vi "new FGGA Serial Data Server & Recordingv4.3.vi"(0 "VISA resource name out":refnum<visa-resource-name>, 11 "error IO":errorcluster) -> ()   [LabVIEW 2014]
uses:
  <vilib>/Platform/TimedLoop/XDataNode/timing_clust.ctl
  <vilib>/Platform/TimedLoop/XDataNode/nitl_modes.ctl
  <vilib>/Platform/TimedLoop/XDataNode/wakeup.ctl
  C:/Program Files (x86)/National Instruments/LabVIEW 2014/examples/Data Communication/Network Streams/Simple Network Streams/support/Network Stream Command.ctl
  <vilib>/Utility/error.llb/whitespace.ctl
  <vilib>/Instr/_visa.llb/VISA Configure Serial Port (Instr).vi
  <vilib>/Utility/tcp.llb/UDP Multicast Write-Only Open.vi
  <vilib>/platform/TimedLoop/XDataNode/XDataNode.xnode
  <vilib>/Platform/TimedLoop/XDataNode/XDNodeRunTimeDep.lvlib
panel:
  out "ASCII_file_out":string
  out "Unix time":u32
  out "FGGA Pump":bool
  out "Flight Number":string
  out "Stop File Write":bool
  out "Default file name":string
  out "MFC":dbl[](array[numeric])
  out "FGGA restart":bool
  out "V4":bool
  out "V3":bool
  out "V2":bool
  out "V1":bool
  out "error out 2":errorcluster
  out "error out":errorcluster
  in  "MFC_1 SLPM set value":dbl
  out "Value Read":string
  out "status":bool
  in  "VISA resource name":refnum<visa-resource-name>="ASRL3::INSTR"
  in  "timeout (10sec) 2":u32=3000
  in  "Clear Display\nErrors":bool
  out "Data Processing":bool
  out "TCP Binary Packet":string
  out "UDP Time Stamp Offset":i32=1
  out "Data String":string
  out "UDP_ACSII_Out":string
  out "Serial error out":errorcluster
  out "SEPTIC TCP Error Out":errorcluster
  out "TCP packet\nSend To SEPTIC":bool
  out "FISH TCP Error Out":errorcluster
  out "TCP packet\nSend To FISH":bool
  out "UDP_Pack_num":u32
  out "UDP_Out Status":bool
  out "UDP_Out_Error Out":errorcluster
  out "Data Array":string[](array[string])
  out "RAW DATA":string
  in  "stop":bool
  out "Number of times \nRead time out":u32
  out "Loop count":i32
  # "Date"
  # "Time"
  # "CH4_wet_ppm"
  # "1"
  # "CO4_wet_ppm_sd"
  # "H2O_ppm"
  # "3"
  # "H2O_ppm_sd"
  # "CO2_wet_ppm"
  # "5"
  # "CO2_wet_ppm_sd"
  # "CH4_dry_ppm"
  # "CH4_dry_ppm_sd"
  # "CO2_dry_ppm"
  # "CO2_dry_ppm_sd"
  # "cell_pressure_torr"
  # "11"
  # "cell_pressure_torr_sd"
  # "13"
  # "cell_temp_degC"
  # "cell_temp_degC_sdev"
  # "ambient(bench)_temp_degC"
  # "15"
  # "ambient(bench)_temp_dedgC_sd"
  # "17"
  # "RDA_us"
  # "RDA_us_sd"
  # "RDB_us"
  # "19"
  # "RDB_us_sd"
  # "Fitflag"
  # "21"
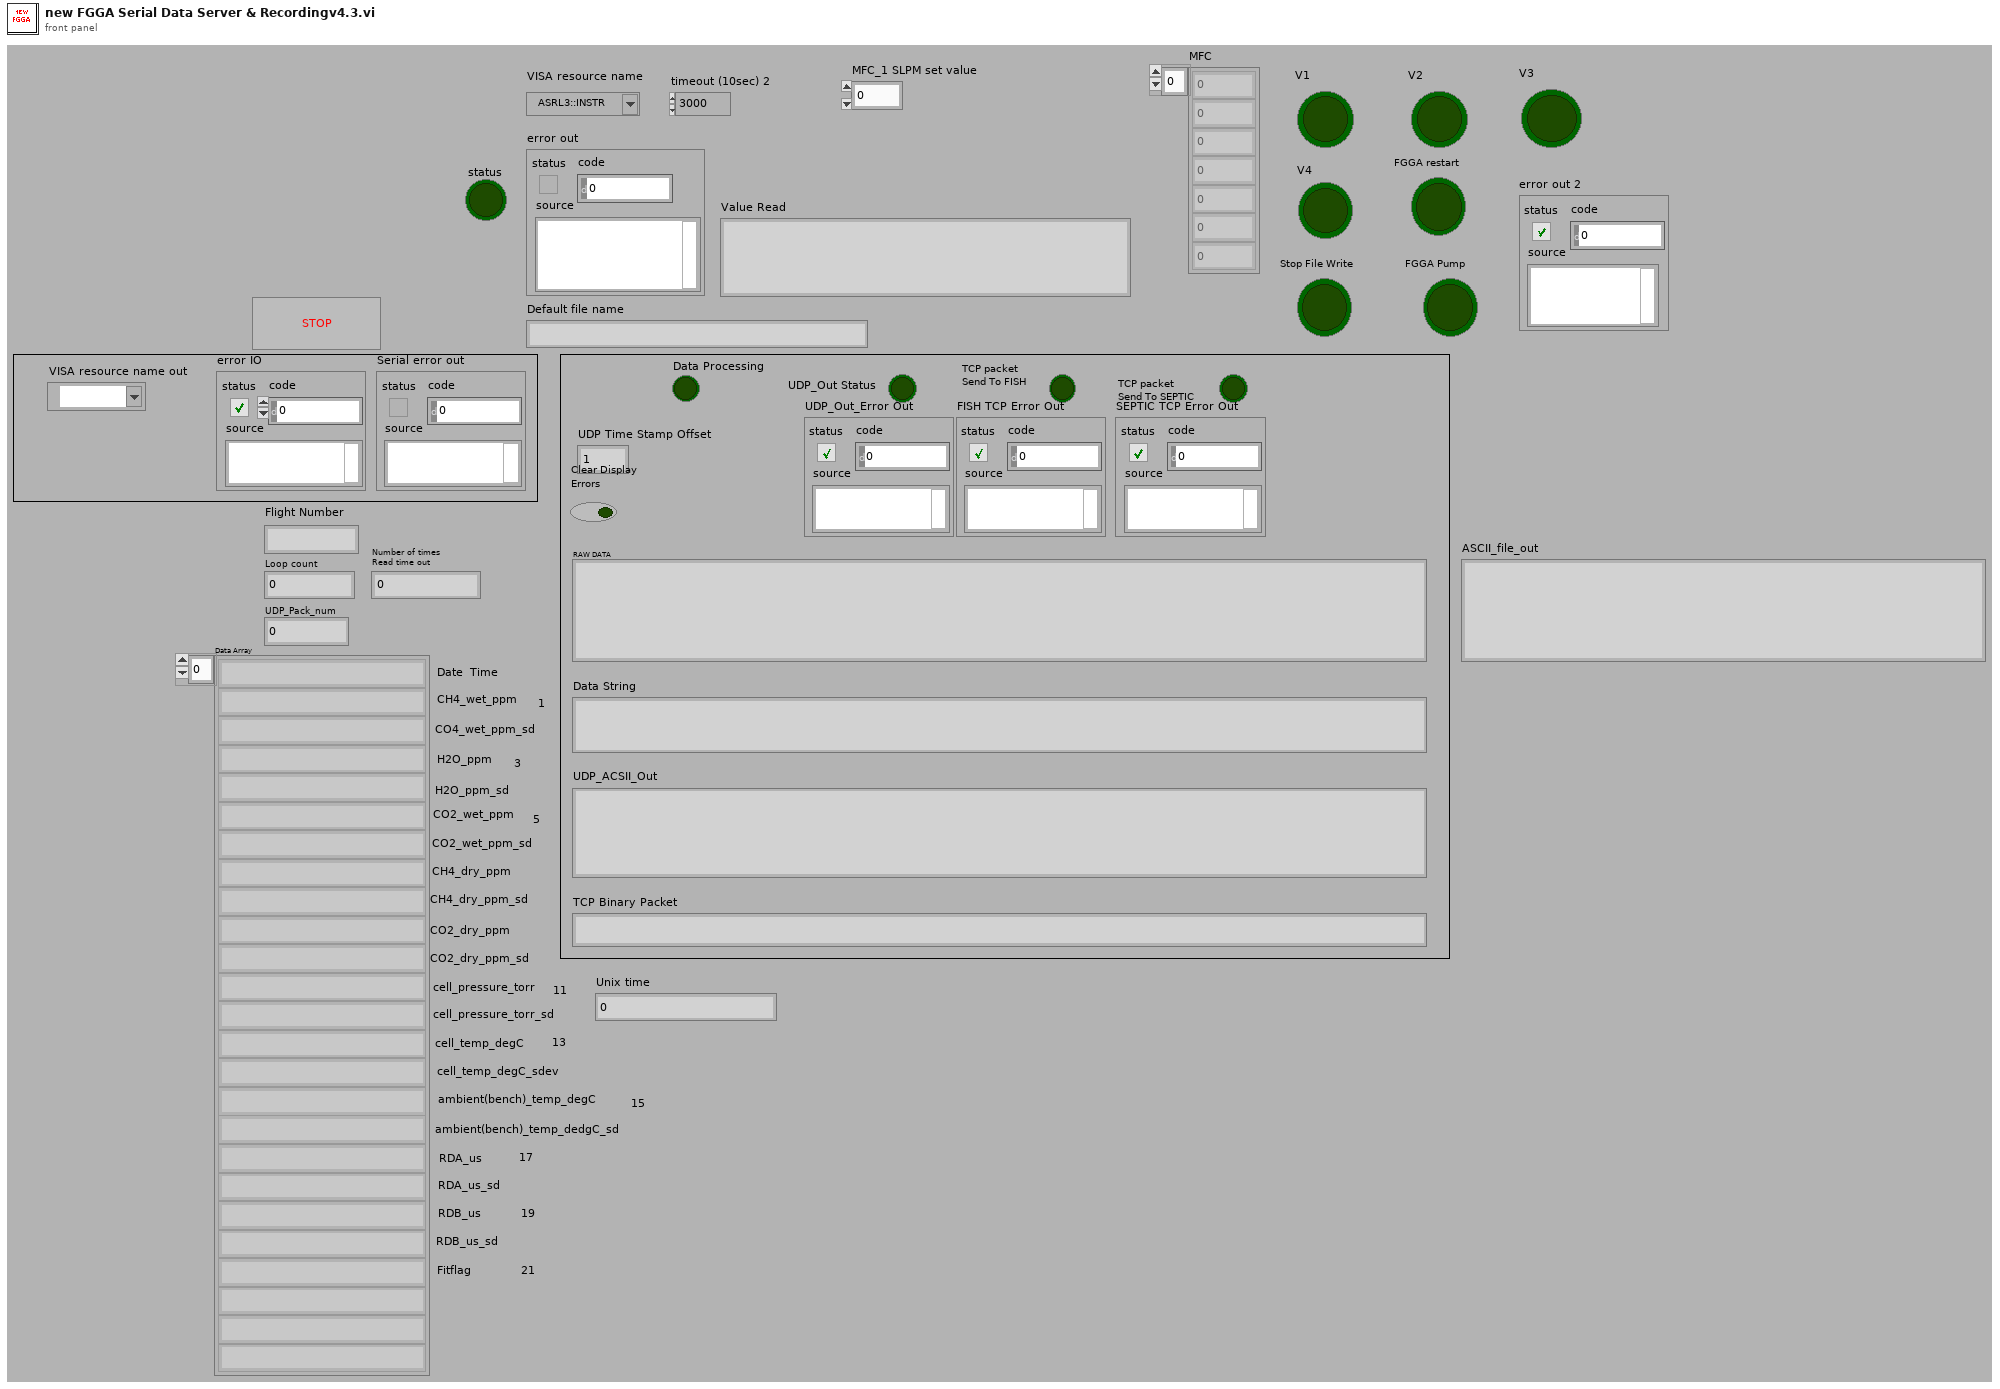
[diagram p1: front panel]
types:
  T1 = typedef "XDNodeRunTimeDep.lvlib/timing_clust.ctl" = cluster{"Expected End [f-1]":u64, "Actual End [f-1]":u64, "Finished Late? [f-1]":bool, "Expected End [i-1]":u64, "Actual End [i-1]":u64, "Finished Late? [i-1]":bool, "Expected Start [i]":u64, "Actual Start [i]":u64, "Expected Start [f]":u64, "Actual Start [f]":u64, "Source Name":string, "Structure Name":string, "Period":i64, "Deadline":i64, "Offset":i64, "Start":i64, "Priority":i32, "Timeout":i32, "Mode":T2, "Wakeup Reason":T3, "Error":errorcluster, "Source Type":string, "Secondary Source Type":string, "Global End Time":u64, "Global Start Time":u64, "Frame Duration":u64, "Iteration Duration":u64, "Assigned CPU":i32, "I/O Scan Engine Mode":u32}
  T2 = typedef "XDNodeRunTimeDep.lvlib/nitl_modes.ctl" = enum32{"No Change", "Process missed periods, maintain original phase", "Discard missed periods, maintain original phase", "Process missed periods, ignore original phase", "Discard missed periods, ignore original phase"}
  T3 = typedef "XDNodeRunTimeDep.lvlib/wakeup.ctl" = enum32{"Normal", "Aborted", "Asynchronous wakeup", "Timing source error", "Timed loop error", "Timeout"}
  T4 = enum16{"open", "replace", "create", "open or create", "replace or create", "replace or create with confirmation"}
  T5 = typedef "Network Stream Command.ctl" = cluster{"Message":string, "Message Data":variant}
  T6 = typedef "whitespace.ctl" = u16
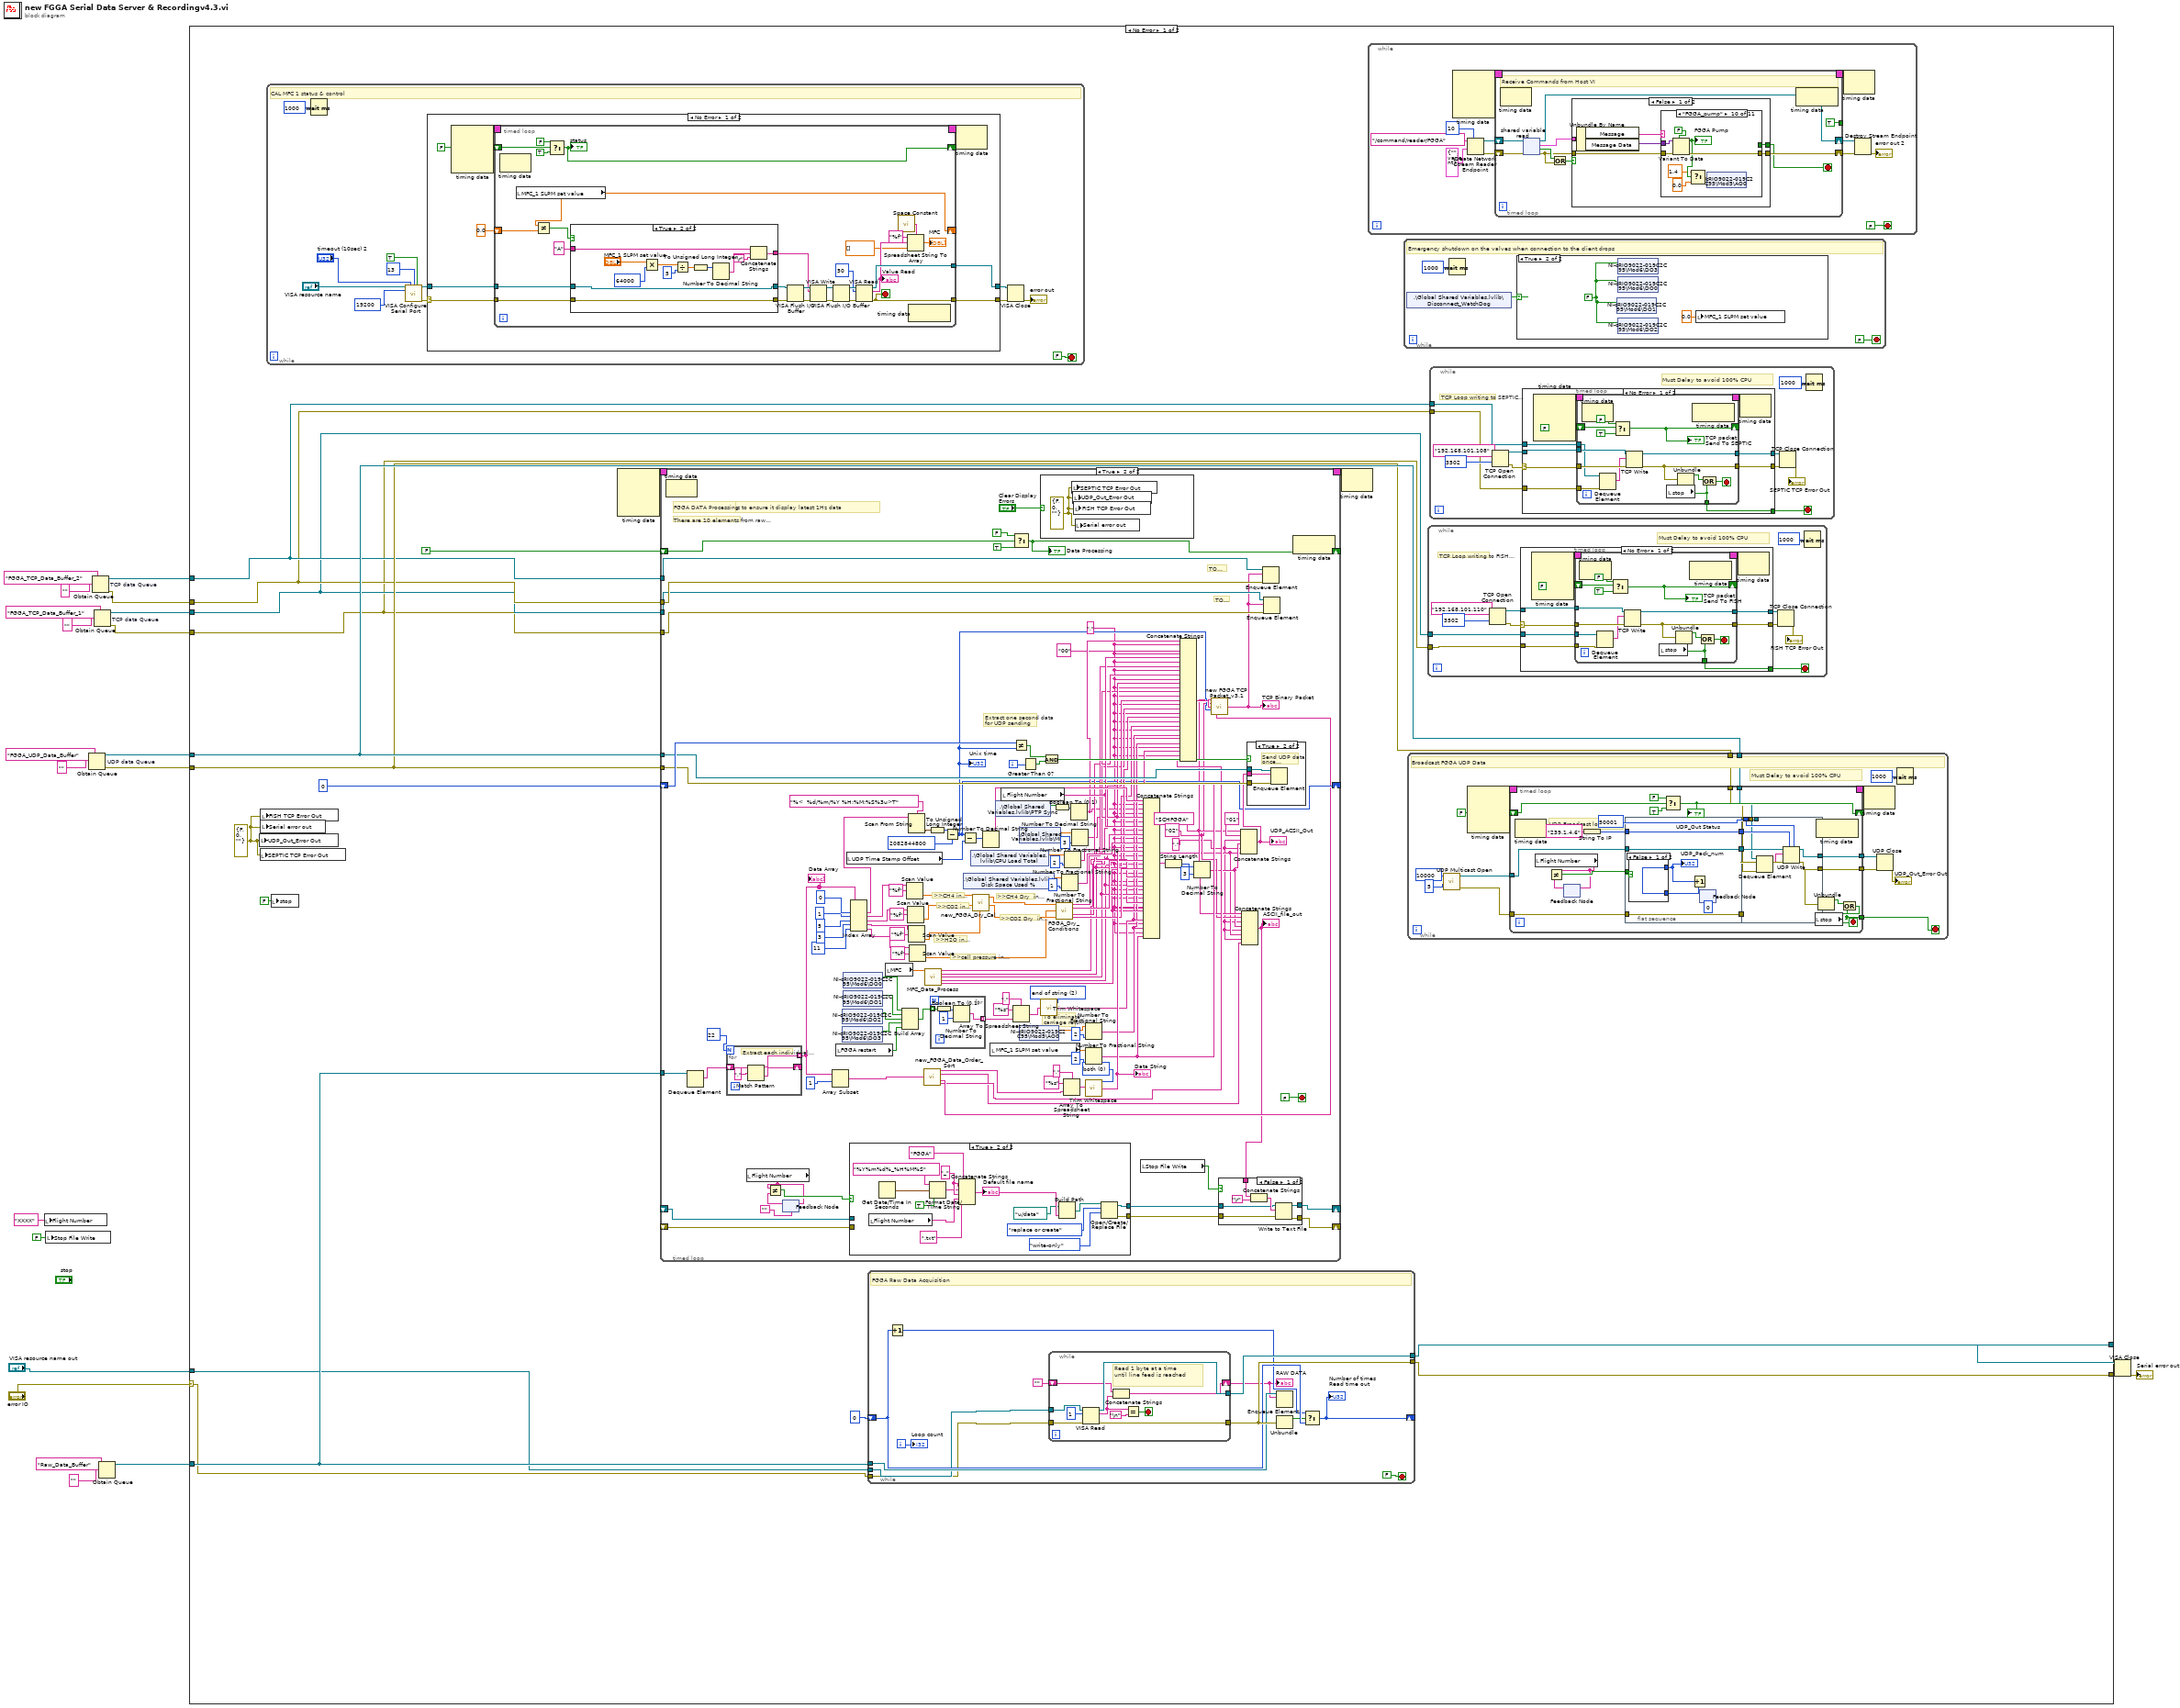
[diagram p0: block diagram]
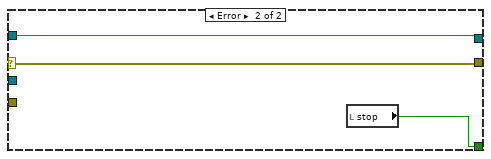
[diagram p2: hidden frame]
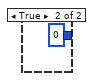
[diagram p3: hidden frame]
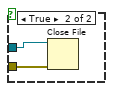
[diagram p5: hidden frame]
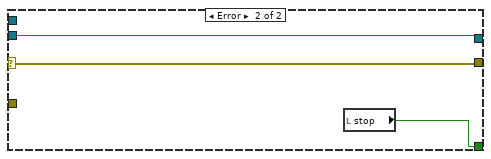
[diagram p8: hidden frame]
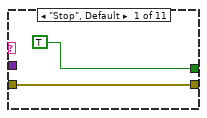
[diagram p10: hidden frame]
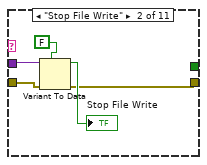
[diagram p11: hidden frame]
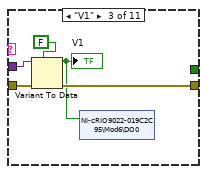
[diagram p12: hidden frame]
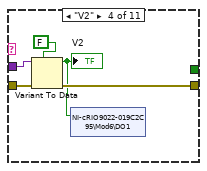
[diagram p13: hidden frame]
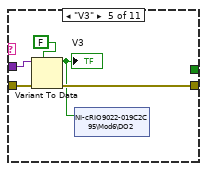
[diagram p14: hidden frame]
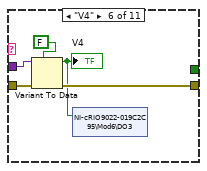
[diagram p15: hidden frame]
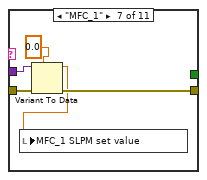
[diagram p16: hidden frame]
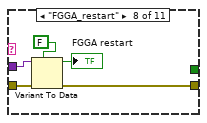
[diagram p17: hidden frame]
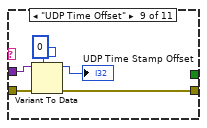
[diagram p18: hidden frame]
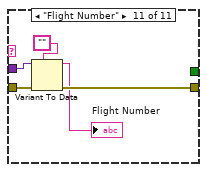
[diagram p19: hidden frame]
diagram:
  n1 = local write "Flight Number"("XXXX" ("Flight Number")) -> ()
  n2 = local write "Stop File Write"(FALSE ("Stop File Write")) -> ()
  n3 = Obtain Queue "UDP data Queue"(name (unnamed)="FGGA_UDP_Data_Buffer", element data type="") -> (queue out=w14:refnum<queue>, error out=w13:errorcluster)  [unwired: 3 in, 1 out]
  n4 = Obtain Queue "TCP data Queue"(name (unnamed)="FGGA_TCP_Data_Buffer_2", element data type="") -> (queue out=w8:refnum<queue>, error out=w7:errorcluster)  [unwired: 3 in, 1 out]
  n5 = Obtain Queue "TCP data Queue"(name (unnamed)="FGGA_TCP_Data_Buffer_1", element data type="") -> (queue out=w6:refnum<queue>, error out=w5:errorcluster)  [unwired: 3 in, 1 out]
  n6 = Obtain Queue(name (unnamed)="Raw_Data_Buffer", element data type="") -> (queue out=w20:refnum<queue>)  [unwired: 3 in, 2 out]
  n7 = case shown="No Error" "error IO" {
    selector: "error IO" -> [w27 w538]
    tunnel: "VISA resource name out" -> [w28 w539]
    tunnel: [w39 w539] -> w17
    tunnel: [w40 w538] -> w18
    tunnel: w20 -> [w38 _]
    tunnel: w14 -> [w36 _]
    tunnel: w13 -> [w35 _]
    tunnel: w8 -> [w34 _]
    tunnel: w7 -> [w33 _]
    tunnel: w6 -> [w32 _]
    tunnel: w5 -> [w31 _]
    frame No Error {
      w24 = errorcluster {"status"=FALSE, "code"=0, "source"=""} ("UDP Error Out")
      n8 = local write "UDP_Out_Error Out"(w24) -> ()
      n9 = local write "SEPTIC TCP Error Out"(w24) -> ()
      n10 = local write "FISH TCP Error Out"(w24) -> ()
      n11 = local write "Serial error out"(w24) -> ()
      n12 = while {
        stop <- FALSE stop-if-true
        # "CAL MFC 1 status & control"
        n13 = Wait (ms)(milliseconds to wait=u32 1000) -> ()  [unwired: 1 out]
        n14 = call-poly "VISA Configure Serial Port"("VISA resource name"="VISA resource name", "timeout (10sec)"="timeout (10sec) 2", "termination char\n(0xA = '\\n' = LF)"=u8 13 ("termination char\n(0xA = '\\n' = LF)"), "Enable Termination\nChar (T)"=TRUE ("Enable Termination\nChar (T)"), "baud rate (9600)"=u32 19200) -> ("VISA resource name out"=w479:refnum<visa-resource-name>, "error out"=w475:errorcluster)  [unwired: 9 in]
        n15 = case shown="No Error" w475 {
          selector: w475 -> [w486 w536]
          tunnel: w479 -> [w487 w537]
          tunnel: [w485 w537] -> w478
          tunnel: [w484 w536] -> w477
          frame No Error {
            n16 = node-c288() -> (w482:T1)  [unwired: 4 in]
            n17 = timed-loop {
              tunnel: w487 -> [w510]
              tunnel: w486 -> [w508]
              tunnel: [w501] -> w485
              tunnel: [w496] -> w484
              shift-right: [w497] -> _
              shift-left: FALSE -> [w500]
              timing: w482 -> [_]
              timing-out: [_] -> w481
              shift-right: [w488] -> _
              shift-left: 0.0 -> [w490]
              stop <- w496 stop-if-true
              n18 = node-c288() -> ()  [unwired: 1 in, 1 out]
              n19 = local read "MFC_1 SLPM set value"() -> (w488:dbl)
              n20 = Not Equal?(x=w488, y=w490) -> (x != y?=w489:bool)
              n21 = Select(t=FALSE, s=w500, f=TRUE) -> (s? t:f=w497:bool)
              "status" <- w497
              n22 = case shown="True" w489 {
                tunnel: w510 -> [w518 w533]
                tunnel: [w518 w533] -> w509
                tunnel: w508 -> [w517 w532]
                tunnel: [w517 w532] -> w507
                tunnel: "A" -> [w521 w525]
                tunnel: [w519 w522] -> w505
                frame False {
                  n23 = Concatenate Strings(w521, "\r") -> (w519:string)
                }
                frame True {
                  n24 = Multiply(x="MFC_1 SLPM set value", y=u32 64000) -> (x*y=w529:dbl)
                  n25 = Divide(x=w529, y=u32 5) -> (x/y=w527:dbl)
                  n26 = To Unsigned Long Integer(number=w527) -> (unsigned 32bit integer=w526:u32)
                  n27 = Number To Decimal String(number=w526) -> (decimal integer string=w524:string)  [unwired: 1 in]
                  n28 = Concatenate Strings(w525, w524, "\r") -> (w522:string)
                }
              }
              n29 = VISA Flush I/O Buffer(VISA resource name=w509, error in (no error)=w507) -> (VISA resource name out=w512:refnum<visa-resource-name>, error out=w511:errorcluster)  [unwired: 1 in]
              n30 = VISA Write(VISA resource name=w512, write buffer=w505, error in (no error)=w511) -> (VISA resource name out=w504:refnum<visa-resource-name>, error out=w503:errorcluster)  [unwired: 1 out]
              n31 = VISA Flush I/O Buffer(VISA resource name=w504, error in (no error)=w503) -> (VISA resource name out=w514:refnum<visa-resource-name>, error out=w513:errorcluster)  [unwired: 1 in]
              n32 = VISA Read(VISA resource name=w514, byte count=u32 50, error in (no error)=w513) -> (VISA resource name out=w501:refnum<visa-resource-name>, read buffer=w495:string, error out=w496:errorcluster)  [unwired: 1 out]
              "Value Read" <- w495
              n33 = call <vilib>:"Space Constant.vi"() -> ("String"=w494:string)
              n34 = Spreadsheet String To Array(delimiter (Tab)=w494, format string="%f", spreadsheet string=w495, array type (2D Dbl)=dbl[] []) -> (array=→"MFC":dbl[])
              n35 = node-c288() -> ()  [unwired: 1 in, 1 out]
            }
            n36 = node-c288(w481) -> ()  [unwired: 1 out]
          }
          frame Error {
          }
        }
        n37 = VISA Close(VISA resource name=w478, error in (no error)=w477) -> (error out=→"error out":errorcluster)
      }
      n38 = local write "stop"(FALSE ("stop")) -> ()
      n39 = node-c288() -> (w26:T1)  [unwired: 4 in]
      n40 = timed-loop {
        timing: w26 -> [_]
        timing-out: [_] -> w25
        tunnel: w38 -> [w290]
        tunnel: w36 -> [w258]
        tunnel: w35 -> [w257]
        shift-right: [w185] -> _
        shift-left: u32 0 -> [w261]
        tunnel: w34 -> [w256]
        tunnel: w33 -> [w255]
        tunnel: w32 -> [w254]
        tunnel: w31 -> [w253]
        shift-right: [w249] -> _
        shift-left: FALSE -> [w252]
        shift-right: [w238] -> _
        shift-left: _ -> [w230]
        shift-right: [w228] -> _
        shift-left: _ -> [w229]
        i -> [w260]
        stop <- FALSE stop-if-true
        w202 = T6 2 items=["both", "start of string", "end of string"] ("location (both)")
        w178 = ","
        w279 = T6 0 items=["both", "start of string", "end of string"] ("location (both)")
        w166 = ","
        w170 = "02"
        w171 = "$CHFGGA"
        # "To eliminate\ncarriage return"
        # ">>cell pressure in torr>>"
        # "There are 10 elements from raw packet"
        # "TO SEPTIC"
        # "TO FISH"
        # "Extract one second data\nfor UDP sending"
        # ">>CO2 Dry  in ppm>>"
        # ">>CH4 Dry  in ppb>>"
        # ">>H2O in ppm>>"
        # ">>CO2 in ppm>>"
        # ">>CH4 in ppm>>"
        # "Loop Time is 500msec to ensure it display latest 1Hz data"
        # "FGGA DATA Processing"
        n41 = node-c288() -> ()  [unwired: 1 in, 1 out]
        n42 = Dequeue Element(queue=w290) -> (element=w248:string)  [unwired: 2 in, 3 out]
        n43 = for {
          N: 22 -> [_]
          shift-right: [w327] -> _
          shift-left: w248 -> [w325]
          tunnel: [w326] -> w284 mode=indexing
          # "Extract each individual param"
          n44 = Match Pattern(string=w325, regular expression=",") -> (before substring=w326:string, after substring=w327:string)  [unwired: 1 in, 2 out]
        }
        "Data Array" <- w284
        n45 = local read "Flight Number"() -> (w227:string)
        n46 = feedback #1("" ("Flight Number")) -> (w235:string)
        n47 = Not Equal?(x=w227, y=w235) -> (x != y?=w233:bool)
        n48 = feedback-in #1(w227) -> ()
        n49 = Array Subset(array=w284, index=1) -> (w176:string[])  [unwired: 1 in]
        n50 = local read "FGGA restart"() -> (w212:bool)
        n51 = shared-variable "NI-cRIO9022-019C2C95\\Mod6\\DO2"() -> (w218:bool)  [unwired: 1 in, 1 out]
        n52 = shared-variable "NI-cRIO9022-019C2C95\\Mod6\\DO3"() -> (w217:bool)  [unwired: 1 in, 1 out]
        n53 = shared-variable "NI-cRIO9022-019C2C95\\Mod6\\DO0"() -> (w220:bool)  [unwired: 1 in, 1 out]
        n54 = shared-variable "NI-cRIO9022-019C2C95\\Mod6\\DO1"() -> (w219:bool)  [unwired: 1 in, 1 out]
        n55 = local read "UDP Time Stamp Offset"() -> (w201:i32)
        n56 = case shown="True" w233 {
          tunnel: [w296 w298] -> w232
          tunnel: [w295 w297] -> w231
          tunnel: w230 -> [w296 _]
          tunnel: w229 -> [w295 _]
          frame False {
          }
          frame True {
            w304 = "_" ("string")
            n57 = local read "Flight Number"() -> (w311:string)
            n58 = Get Date/Time In Seconds() -> (seconds since 1Jan1904=w299:timestamp)
            n59 = Format Date/Time String(time format string (%c)="%Y%m%d%_%H%M%S", seconds (now)=w299, UTC format=TRUE) -> (date/time string=w301:string)
            n60 = Concatenate Strings("FGGA" ("string"), w304, w301, w304, w311, ".txt" ("string")) -> (w306:string)
            "Default file name" <- w306
            n61 = Build Path(base path=path "u:/data", name or relative path=w306) -> (appended path=w310:path)
            n62 = Open/Create/Replace File(file path (use dialog)=w310, operation (0:open)=T4."replace or create", access (0:read/write)=enum16{"read/write", "read-only", "write-only"}."write-only") -> (refnum out=w298:refnum<file>, error out=w297:errorcluster)  [unwired: 3 in, 1 out]
          }
        }
        n63 = Index Array(array=w284, index #1=0 ("index"), index #2=1 ("index"), index #3=5 ("index"), index #4=3 ("index"), index #5=11 ("index")) -> (element #1=w179:string, element #2=w184:string, element #3=w183:string, element #4=w182:string, element #5=w181:string)
        n64 = local read "MFC"() -> (w239:dbl[])
        n65 = Build Array(w220, w219, w218, w217, w212) -> (w216:bool[])
        n66 = Scan Value(string=w184, format string="%f") -> (value=w270:dbl)  [unwired: 1 in, 1 out]
        n67 = Scan Value(string=w183, format string="%f") -> (value=w269:dbl)  [unwired: 1 in, 1 out]
        n68 = Scan From String(format string="%<  %d/%m/%Y %H:%M:%S%3u>T", input string=w179) -> (output 1=w266:timestamp)  [unwired: 3 in, 3 out]
        n69 = Scan Value(string=w182, format string="%f") -> (value=w240:dbl)  [unwired: 1 in, 1 out]
        n70 = Scan Value(string=w181, format string="%f") -> (value=w241:dbl)  [unwired: 1 in, 1 out]
        n71 = call "new_FGGA_Data_Order_Sort.vi"("Data In"=w176) -> ("UDP Data Out"=w175:string[], "ASCII Ambient(bench)_temp"=w165:string, "TCP Data Out"=w174:string[], "TCP Ambient(bench)_temp"=w173:string)  [unwired: 11 in]
        n72 = call "MFC_Data_Process.vi"("MFC"=w239) -> ("MFC Absolute Pressure"=w196:string, "MFC Temperature"=w195:string, "MFC Volumetric Flow"=w194:string, "MFC Mass Flow"=w193:string, "MFC Set Point"=w192:string)  [unwired: 10 in]
        n73 = To Unsigned Long Integer(number=w266) -> (unsigned 32bit integer=w267:u32)
        n74 = for {
          tunnel: w216 -> [w293] mode=indexing
          tunnel: [w292] -> w213 mode=indexing
          n75 = Boolean To (0,1)(Boolean=w293) -> (0, 1=w294:i16)
          n76 = Number To Decimal String(number=w294, width (-)=i16 1) -> (decimal integer string=w292:string)
        }
        n77 = Subtract(x=w267, y=u32 2082844800) -> (x-y=w185:u32)
        "Unix time" <- w185
        n78 = Subtract(x=w185, y=w201) -> (x-y=w264:u32)
        n79 = shared-variable ".\\Global Shared Variables.lvlib\\Disk Space Used %"() -> (w205:dbl)  [unwired: 1 in, 1 out]
        n80 = shared-variable ".\\Global Shared Variables.lvlib\\CPU Load Total"() -> (w226:dbl)  [unwired: 1 in, 1 out]
        n81 = call "new_FGGA_Dry_Cal.vi"("H2O"=w240, "CO2_Wet"=w269, "CH4_Wet"=w270) -> ("CO2_Dry"=w243:dbl, "CH4_Dry"=w245:dbl)  [unwired: 7 in]
        n82 = Number To Decimal String(number=w264) -> (decimal integer string=w265:string)  [unwired: 1 in]
        n83 = local read "MFC_1 SLPM set value"() -> (w208:dbl)
        n84 = shared-variable ".\\Global Shared Variables.lvlib\\PTP Sync"() -> (w221:bool)  [unwired: 1 in, 1 out]
        n85 = local read "Flight Number"() -> (w200:string)
        n86 = Array To Spreadsheet String(delimiter (Tab)=",", array=w213, 3:"%s" ("format string")) -> (spreadsheet string=w203:string)
        n87 = Select(t=FALSE, s=w252, f=TRUE) -> (s? t:f=w249:bool)
        "Data Processing" <- w249
        n88 = Not Equal?(x=w261, y=w185) -> (x != y?=w262:bool)
        n89 = shared-variable ".\\Global Shared Variables.lvlib\\MFM"() -> (w224:dbl)  [unwired: 1 in, 1 out]
        n90 = shared-variable "NI-cRIO9022-019C2C95\\Mod5\\AO0"() -> (w210:dbl)  [unwired: 1 in, 1 out]
        n91 = Greater Than 0?(x=w260) -> (x > 0?=w263:bool)
        n92 = case shown="True" "Clear Display\nErrors" {
          frame False {
          }
          frame True {
            w321 = errorcluster {"status"=FALSE, "code"=0, "source"=""} ("UDP Error Out")
            n93 = local write "SEPTIC TCP Error Out"(w321) -> ()
            n94 = local write "UDP_Out_Error Out"(w321) -> ()
            n95 = local write "FISH TCP Error Out"(w321) -> ()
            n96 = local write "Serial error out"(w321) -> ()
          }
        }
        n97 = call <vilib>:"Trim Whitespace.vi"("string"=w203, "location (both)"=w202) -> ("trimmed string"=w191:string)
        n98 = Compound Arithmetic op=AND(w262, w263) -> (w259:bool)
        n99 = Boolean To (0,1)(Boolean=w221) -> (0, 1=w222:i16)
        n100 = call "FGGA_Dry_Conditions.vi"("CH4_Dry"=w245, "Pressure"=w241, "CO2_Dry"=w243) -> ("CH4_Dry_TCP"=w199:string, "CH4_Dry_UDP"=w247:string, "CO2_Dry_TCP"=w198:string, "CO2_Dry_UDP"=w246:string)  [unwired: 9 in]
        n101 = Number To Fractional String(number=w205, precision (6)=i16 1) -> (F-format string=w204:string)  [unwired: 2 in]
        n102 = Array To Spreadsheet String(delimiter (Tab)=",", array=w175, 3:"%s" ("format string")) -> (spreadsheet string=w278:string)
        n103 = Number To Fractional String(number=w226, precision (6)=i16 2) -> (F-format string=w207:string)  [unwired: 2 in]
        n104 = Number To Decimal String(number=w222) -> (decimal integer string=w187:string)  [unwired: 1 in]
        n105 = Number To Fractional String(number=w224, precision (6)=i16 3) -> (F-format string=w197:string)  [unwired: 2 in]
        n106 = Number To Fractional String(number=w210, precision (6)=i16 2) -> (F-format string=w190:string)  [unwired: 2 in]
        n107 = Number To Fractional String(number=w208, precision (6)=i16 2) -> (F-format string=w189:string)  [unwired: 2 in]
        n108 = call <vilib>:"Trim Whitespace.vi"("string"=w278, "location (both)"=w279) -> ("trimmed string"=w277:string)
        "Data String" <- w277
        n109 = local read "Stop File Write"() -> (w236:bool)
        n110 = Concatenate Strings(w265, w178, w187, w178, w197, w178, w200, w178, w207, w178, w204, w178, w277, w178, w247, w178, w246, w178, w196, w178, w195, w178, w194, w178, w193, w178, w192, w178, w191, w178, w190, w178, w189) -> (w168:string)
        n111 = String Length(string=w168) -> (length=w287:i32)
        n112 = Concatenate Strings(w187, w178, "00", w178, w200, w178, w199, w178, w198, w178, w197, w178, w196, w178, w195, w178, w194, w178, w193, w178, w192, w178, w191, w178, w190, w178, w189, w178, w173) -> (w188:string)
        n113 = Number To Decimal String(number=w287, width (-)=i16 3) -> (decimal integer string=w169:string)
        n114 = call "new FGGA TCP Packet_v3.1.vi"("ID"=w171, "Version"=w170, "TCP Packet In"=w188, "utc_time"=w185, "Data Array"=w174) -> ("TCP Binary Packet"=w177:string)  [unwired: 10 in]
        "TCP Binary Packet" <- w177
        n115 = Concatenate Strings(w171, "01", w166, w169, w166, w168) -> (w237:string)
        "UDP_ACSII_Out" <- w237
        n116 = Concatenate Strings(w171, w170, w166, w169, w166, w168, w166, w165) -> (w167:string)
        "ASCII_file_out" <- w167
        n117 = case shown="False" w236 {
          tunnel: w167 -> [w318 _]
          tunnel: [w315 _] -> w238
          tunnel: w232 -> [w314 w320]
          tunnel: w231 -> [w313 w319]
          tunnel: [w312 _] -> w228
          frame False {
            n118 = Concatenate Strings(w318, "\r") -> (w316:string)
            n119 = Write to Text File(file (use dialog)=w314, text=w316, error in=w313) -> (refnum out=w315:refnum<file>, error out=w312:errorcluster)  [unwired: 2 out]
          }
          frame True {
            n120 = Close File(refnum=w320, error in=w319) -> ()  [unwired: 2 out]
          }
        }
        n121 = case shown="True" w259 {
          tunnel: w237 -> [_ w324]
          tunnel: w258 -> [_ w323]
          tunnel: w257 -> [_ w322]
          frame False {
          }
          frame True {
            # "Send UDP data once\na second"
            n122 = Enqueue Element(queue=w323, element=w324, error in (no error)=w322) -> ()  [unwired: 1 in, 3 out]
          }
        }
        n123 = Enqueue Element(queue=w256, element=w177, error in (no error)=w255) -> ()  [unwired: 1 in, 3 out]
        n124 = Enqueue Element(queue=w254, element=w177, error in (no error)=w253) -> ()  [unwired: 1 in, 3 out]
        n125 = node-c288() -> ()  [unwired: 1 in, 1 out]
      }
      n126 = while {
        tunnel: w28 -> [w42]
        tunnel: w27 -> [w41]
        tunnel: [w53] -> w40
        shift-right: [w49] -> _
        shift-left: u32 0 -> [w50]
        tunnel: [w52] -> w39
        tunnel: w38 -> [w47]
        i -> [w51]
        stop <- FALSE stop-if-true
        # "FGGA Raw Data Acquisition"
        n127 = Increment(x=w50) -> (x+1=w48:u32)
        n128 = while {
          tunnel: [w63] -> w52
          tunnel: [w62] -> w53
          tunnel: w42 -> [w61]
          tunnel: w41 -> [w60]
          shift-right: [w58] -> w44
          shift-left: "" -> [w59]
          stop <- w55 stop-if-true
          # "Read 1 byte at a time \nuntil line feed is reached"
          n129 = VISA Read(VISA resource name=w61, byte count=u32 1, error in (no error)=w60) -> (VISA resource name out=w63:refnum<visa-resource-name>, read buffer=w57:string, error out=w62:errorcluster)  [unwired: 1 out]
          n130 = Concatenate Strings(w59, w57) -> (w58:string)
          n131 = Equal?(x=w57, y="\n") -> (x = y?=w55:bool)
        }
        "RAW DATA" <- w44
        n132 = Enqueue Element(queue=w47, element=w44) -> ()  [unwired: 2 in, 3 out]
        n133 = Unbundle(w53) -> ("status"=w46:bool)  [unwired: 2 out]
        n134 = Select(t=w48, s=w46, f=w50) -> (s? t:f=w49:u32)
        "Number of times \nRead time out" <- w49
        "Loop count" <- w51
      }
      n135 = node-c288(w25) -> ()  [unwired: 1 out]
      n136 = while {
        stop <- FALSE stop-if-true
        n137 = node-c288() -> (w381:T1)  [unwired: 4 in]
        n138 = Create Network Stream Reader Endpoint(7:10 ("reader buffer size"), 9:T5 {"Message"="", "Message Data"=variant} ("Message Cluster"), 11:"/command/reader/FGGA" ("reader url")) -> (0:w386:errorcluster, 3:w387:refnum<k21>)  [unwired: 4 in]
        n139 = timed-loop "Host->Target Command Reader" {
          shift-right: [w397] -> w384
          shift-left: w386 -> [w400]
          shift-right: [w398] -> w383
          shift-left: w387 -> [w399]
          tunnel: [TRUE] -> _
          timing: w381 -> [_]
          timing-out: [_] -> w380
          stop <- w391 stop-if-true
          # "Receive Commands from Host VI"
          n140 = node-c288() -> ()  [unwired: 1 in, 1 out]
          n141 = shared-variable-read(w399, w400) -> (w398:refnum<k21>, w393:errorcluster, w395:bool, w396:T5)  [unwired: 1 in]
          n142 = Or(x=w395, y=w393) -> (x .or. y?=w394:bool)
          n143 = case shown="False" w394 {
            selector: w394 -> [_ w464]
            tunnel: w393 -> [w408 w465]
            tunnel: [w407 w465] -> w397
            tunnel: w396 -> [w405 _]
            tunnel: [w406 w464] -> w391
            frame False {
              n144 = Unbundle By Name(w405) -> ("Message"=w404:string, "Message Data"=w403:variant)
              n145 = case shown="\"FGGA_pump\"" w404 {
                tunnel: w408 -> [w410 w415 w420 w425 w430 w435 w440 w445 w450 w458 w463]
                tunnel: [w410 w411 w419 w424 w429 w434 w439 w444 w449 w457 w462] -> w407
                tunnel: w403 -> [_ w414 w418 w423 w428 w433 w438 w443 w448 w456 w461]
                tunnel: [TRUE _ _ _ _ _ _ _ _ _ _] -> w406
                frame "Stop", Default {
                }
                frame "Stop File Write" {
                  n146 = Variant To Data(error in=w415, type=FALSE, Variant=w414) -> (data=→"Stop File Write":bool, error out=w411:errorcluster)
                }
                frame "V1" {
                  n147 = Variant To Data(error in=w420, type=FALSE, Variant=w418) -> (data=w416:bool, error out=w419:errorcluster)
                  "V1" <- w416
                  n148 = shared-variable "NI-cRIO9022-019C2C95\\Mod6\\DO0"(w416) -> ()  [unwired: 1 in, 1 out]
                }
                frame "V2" {
                  n149 = Variant To Data(error in=w425, type=FALSE, Variant=w423) -> (data=w421:bool, error out=w424:errorcluster)
                  "V2" <- w421
                  n150 = shared-variable "NI-cRIO9022-019C2C95\\Mod6\\DO1"(w421) -> ()  [unwired: 1 in, 1 out]
                }
                frame "V3" {
                  n151 = Variant To Data(error in=w430, type=FALSE, Variant=w428) -> (data=w426:bool, error out=w429:errorcluster)
                  "V3" <- w426
                  n152 = shared-variable "NI-cRIO9022-019C2C95\\Mod6\\DO2"(w426) -> ()  [unwired: 1 in, 1 out]
                }
                frame "V4" {
                  n153 = Variant To Data(error in=w435, type=FALSE, Variant=w433) -> (data=w431:bool, error out=w434:errorcluster)
                  "V4" <- w431
                  n154 = shared-variable "NI-cRIO9022-019C2C95\\Mod6\\DO3"(w431) -> ()  [unwired: 1 in, 1 out]
                }
                frame "MFC_1" {
                  n155 = Variant To Data(error in=w440, type=0.0, Variant=w438) -> (data=w436:dbl, error out=w439:errorcluster)
                  n156 = local write "MFC_1 SLPM set value"(w436) -> ()
                }
                frame "FGGA_restart" {
                  n157 = Variant To Data(error in=w445, type=FALSE, Variant=w443) -> (data=→"FGGA restart":bool, error out=w444:errorcluster)
                }
                frame "UDP Time Offset" {
                  n158 = Variant To Data(error in=w450, type=0, Variant=w448) -> (data=→"UDP Time Stamp Offset":i32, error out=w449:errorcluster)
                }
                frame "FGGA_pump" {
                  n159 = Variant To Data(error in=w458, type=FALSE, Variant=w456) -> (data=w453:bool, error out=w457:errorcluster)
                  "FGGA Pump" <- w453
                  n160 = Select(t=1.4 ("f"), s=w453, f=0.0 ("t")) -> (s? t:f=w454:dbl)
                  n161 = shared-variable "NI-cRIO9022-019C2C95\\Mod5\\AO0"(w454) -> ()  [unwired: 1 in, 1 out]
                }
                frame "Flight Number" {
                  n162 = Variant To Data(error in=w463, type="", Variant=w461) -> (data=→"Flight Number":string, error out=w462:errorcluster)
                }
              }
            }
            frame True {
            }
          }
          n163 = node-c288() -> ()  [unwired: 1 in, 1 out]
        }
        n164 = node-c288(w380) -> ()  [unwired: 1 out]
        n165 = Destroy Stream Endpoint(8:w384, 11:w383) -> (0:→"error out 2":errorcluster)
      }
      n166 = while {
        stop <- FALSE stop-if-true
        # "Emergency shutdown on the valves when connection to the client drops"
        n167 = shared-variable ".\\Global Shared Variables.lvlib\\Disconnect_WatchDog"() -> (w375:bool)  [unwired: 1 in, 1 out]
        n168 = Wait (ms)(milliseconds to wait=u32 1000) -> ()  [unwired: 1 out]
        n169 = case shown="True" w375 {
          frame False {
          }
          frame True {
            w379 = FALSE
            n170 = shared-variable "NI-cRIO9022-019C2C95\\Mod6\\DO1"(w379) -> ()  [unwired: 1 in, 1 out]
            n171 = shared-variable "NI-cRIO9022-019C2C95\\Mod6\\DO3"(w379) -> ()  [unwired: 1 in, 1 out]
            n172 = shared-variable "NI-cRIO9022-019C2C95\\Mod6\\DO0"(w379) -> ()  [unwired: 1 in, 1 out]
            n173 = shared-variable "NI-cRIO9022-019C2C95\\Mod6\\DO2"(w379) -> ()  [unwired: 1 in, 1 out]
            n174 = local write "MFC_1 SLPM set value"(0.0 ("MFC_1 SLPM set value")) -> ()
          }
        }
      }
      n175 = while {
        tunnel: w36 -> [w108]
        tunnel: w35 -> [w107]
        stop <- w109 stop-if-true
        # "Must Delay to avoid 100% CPU"
        # "Broadcast FGGA UDP Data"
        n176 = call-poly <vilib>:"UDP Multicast Open.vi"("time-to-live (1)"=u16 5, "port"=u16 10000) -> ("error out"=w116:errorcluster, "connection ID"=w117:refnum<k16>)  [unwired: 8 in]
        n177 = node-c288() -> (w119:T1)  [unwired: 4 in]
        n178 = timed-loop {
          tunnel: w117 -> [w140]
          tunnel: w116 -> [w139]
          timing: w119 -> [_]
          timing-out: [_] -> w118
          shift-right: [w128] -> _
          shift-left: FALSE -> [w131]
          tunnel: [w127] -> w111
          tunnel: [w125] -> w110
          tunnel: [w123] -> w109
          tunnel: w108 -> [w121]
          tunnel: w107 -> [w120]
          stop <- w124 stop-if-true
          # "UDP Broadcast loop"
          n179 = node-c288() -> ()  [unwired: 1 in, 1 out]
          n180 = local read "Flight Number"() -> (w122:string)
          n181 = feedback-in #2(w122) -> ()
          n182 = feedback #2() -> (w133:string)  [unwired: 1 in]
          n183 = Not Equal?(x=w122, y=w133) -> (x != y?=w132:bool)
          n184 = String To IP(1:"239.1.4.6" ("name")) -> (0:w137:u32)
          n185 = flat-sequence {
            tunnel: w137 -> [w147]
            tunnel: w139 -> [w148]
            tunnel: w140 -> [w149]
            tunnel: [w149] -> w136
            tunnel: [w148] -> w135
            tunnel: [w147] -> w134
            tunnel: w132 -> [w146]
            tunnel: u16 50001 ("port or service name") -> [w160]
            tunnel: w136 -> [w159]
            tunnel: w135 -> [w158]
            tunnel: w134 -> [w157]
            tunnel: [w156] -> w127
            tunnel: [w155] -> w125
            tunnel: w121 -> [w153]
            tunnel: w120 -> [w152]
            frame #0 {
              n186 = feedback #3(u32 0) -> (w143:u32)
              n187 = case shown="False" w146 {
                tunnel: w143 -> [w150 _]
                tunnel: [w150 u32 0] -> w142
                frame False {
                }
                frame True {
                }
              }
              "UDP_Pack_num" <- w142
              n188 = Increment(x=w142) -> (x+1=w144:u32)
              n189 = feedback-in #3(w144) -> ()
            }
            frame #1 {
              n190 = Dequeue Element(queue=w153, error in (no error)=w152) -> (element=w154:string)  [unwired: 1 in, 3 out]
              n191 = UDP Write(address=w157, port or service name=w160, connection ID=w159, data in=w154, 8:w158) -> (error out=w155:errorcluster, 3:w156:refnum<k16>)  [unwired: 1 in]
            }
          }
          n192 = Select(t=FALSE, s=w131, f=TRUE) -> (s? t:f=w128:bool)
          "UDP_Out Status" <- w128
          n193 = local read "stop"() -> (w123:bool)
          n194 = node-c288() -> ()  [unwired: 1 in, 1 out]
          n195 = Unbundle(w125) -> ("status"=w126:bool)  [unwired: 2 out]
          n196 = Compound Arithmetic op=OR(w126, w123) -> (w124:bool)
        }
        n197 = node-c288(w118) -> ()  [unwired: 1 out]
        n198 = UDP Close(connection ID=w111, 8:w110) -> (error out=→"UDP_Out_Error Out":errorcluster)  [unwired: 1 out]
        n199 = Wait (ms)(milliseconds to wait=u32 1000) -> ()  [unwired: 1 out]
      }
      n200 = while {
        tunnel: w32 -> [w66]
        tunnel: w31 -> [w65]
        stop <- w69 stop-if-true
        # "Must Delay to avoid 100% CPU"
        # "TCP Loop writing to FISH Tank"
        n201 = TCP Open Connection(address="192.168.101.110", remote port or service name=u16 3502) -> (connection ID=w72:refnum<k5>, error out=w67:errorcluster)  [unwired: 3 in]
        n202 = case shown="No Error" w67 {
          selector: w67 -> [w77 w104]
          tunnel: w72 -> [w82 w105]
          tunnel: [w81 w105] -> w71
          tunnel: [w80 w104] -> w70
          tunnel: [w79 w103] -> w69
          tunnel: w66 -> [w76 _]
          tunnel: w65 -> [w75 _]
          frame No Error {
            n203 = node-c288() -> (w84:T1)  [unwired: 4 in]
            n204 = timed-loop {
              tunnel: w82 -> [w98]
              tunnel: w77 -> [w97]
              tunnel: [w96] -> w81
              tunnel: [w95] -> w80
              tunnel: [w87] -> w79
              shift-right: [w89] -> _
              shift-left: FALSE -> [w92]
              timing: w84 -> [_]
              timing-out: [_] -> w83
              tunnel: w76 -> [w86]
              tunnel: w75 -> [w85]
              stop <- w93 stop-if-true
              n205 = node-c288() -> ()  [unwired: 1 in, 1 out]
              n206 = Dequeue Element(queue=w86, error in (no error)=w85) -> (element=w88:string)  [unwired: 1 in, 3 out]
              n207 = Select(t=FALSE, s=w92, f=TRUE) -> (s? t:f=w89:bool)
              "TCP packet\nSend To FISH" <- w89
              n208 = TCP Write(connection ID=w98, data in=w88, error in (no error)=w97) -> (connection ID out=w96:refnum<k5>, error out=w95:errorcluster)  [unwired: 1 in, 1 out]
              n209 = local read "stop"() -> (w87:bool)
              n210 = Unbundle(w95) -> ("status"=w94:bool)  [unwired: 2 out]
              n211 = node-c288() -> ()  [unwired: 1 in, 1 out]
              n212 = Compound Arithmetic op=OR(w94, w87) -> (w93:bool)
            }
            n213 = node-c288(w83) -> ()  [unwired: 1 out]
          }
          frame Error {
            n214 = local read "stop"() -> (w103:bool)
          }
        }
        n215 = TCP Close Connection(connection ID=w71, error in (no error)=w70) -> (error out=→"FISH TCP Error Out":errorcluster)  [unwired: 1 in, 1 out]
        n216 = Wait (ms)(milliseconds to wait=u32 1000) -> ()  [unwired: 1 out]
      }
      n217 = while {
        tunnel: w34 -> [w335]
        tunnel: w33 -> [w334]
        stop <- w338 stop-if-true
        # "Must Delay to avoid 100% CPU"
        # "TCP Loop writing to SEPTIC Tank"
        n218 = TCP Open Connection(address="192.168.101.108", remote port or service name=u16 3502) -> (connection ID=w341:refnum<k5>, error out=w336:errorcluster)  [unwired: 3 in]
        n219 = case shown="No Error" w336 {
          selector: w336 -> [w346 w373]
          tunnel: w341 -> [w351 w374]
          tunnel: [w350 w374] -> w340
          tunnel: [w349 w373] -> w339
          tunnel: [w348 w372] -> w338
          tunnel: w335 -> [w345 _]
          tunnel: w334 -> [w344 _]
          frame No Error {
            n220 = node-c288() -> (w353:T1)  [unwired: 4 in]
            n221 = timed-loop {
              tunnel: w351 -> [w367]
              tunnel: w346 -> [w366]
              tunnel: [w365] -> w350
              tunnel: [w364] -> w349
              tunnel: [w356] -> w348
              shift-right: [w358] -> _
              shift-left: FALSE -> [w361]
              timing: w353 -> [_]
              timing-out: [_] -> w352
              tunnel: w345 -> [w355]
              tunnel: w344 -> [w354]
              stop <- w362 stop-if-true
              n222 = node-c288() -> ()  [unwired: 1 in, 1 out]
              n223 = Dequeue Element(queue=w355, error in (no error)=w354) -> (element=w357:string)  [unwired: 1 in, 3 out]
              n224 = Select(t=FALSE, s=w361, f=TRUE) -> (s? t:f=w358:bool)
              "TCP packet\nSend To SEPTIC" <- w358
              n225 = TCP Write(connection ID=w367, data in=w357, error in (no error)=w366) -> (connection ID out=w365:refnum<k5>, error out=w364:errorcluster)  [unwired: 1 in, 1 out]
              n226 = local read "stop"() -> (w356:bool)
              n227 = Unbundle(w364) -> ("status"=w363:bool)  [unwired: 2 out]
              n228 = node-c288() -> ()  [unwired: 1 in, 1 out]
              n229 = Compound Arithmetic op=OR(w363, w356) -> (w362:bool)
            }
            n230 = node-c288(w352) -> ()  [unwired: 1 out]
          }
          frame Error {
            n231 = local read "stop"() -> (w372:bool)
          }
        }
        n232 = TCP Close Connection(connection ID=w340, error in (no error)=w339) -> (error out=→"SEPTIC TCP Error Out":errorcluster)  [unwired: 1 in, 1 out]
        n233 = Wait (ms)(milliseconds to wait=u32 1000) -> ()  [unwired: 1 out]
      }
    }
    frame Error {
    }
  }
  n234 = VISA Close(VISA resource name=w17, error in (no error)=w18) -> (error out=→"Serial error out":errorcluster)
